vi "Enqueue.vi"(7 "Priority (F)":bool, 8 "错误输入（无错误）":errorcluster, 9 "Message Data":variant, 10 "Message":string, 11 "MessageQueue":refnum<queue>) -> (0 "error out":errorcluster, 3 "MessageQueue":refnum<queue>)   [LabVIEW 2019, in "module.lvlib"]
uses:
  module.lvlib
  Message.ctl
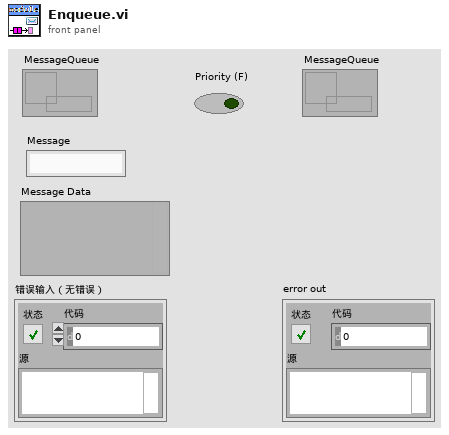
[diagram p1: front panel]
types:
  T1 = typedef "module.lvlib/Message.ctl" = cluster{"Message":string, "Message Data":variant}
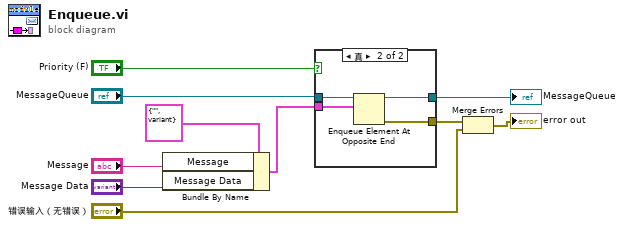
[diagram p0: block diagram]
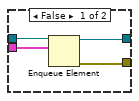
[diagram p2: hidden frame]
diagram:
  n1 = Bundle By Name(cluster=T1 {"Message"="", "Message Data"=variant} ("Message"), "Message"="Message", "Message Data"="Message Data") -> (w3:T1)
  n2 = case shown="真" "Priority (F)" {
    tunnel: "MessageQueue" -> [w14 w18]
    tunnel: [w12 w17] -> w7
    tunnel: [w13 w16] -> w9
    tunnel: w3 -> [w11 w15]
    frame False {
      n3 = Enqueue Element(queue=w14, element=w11) -> (queue out=w12:refnum<queue>, error out=w13:errorcluster)  [unwired: 2 in, 1 out]
    }
    frame True {
      n4 = Enqueue Element At Opposite End(queue=w18, element=w15) -> (queue out=w17:refnum<queue>, error out=w16:errorcluster)  [unwired: 2 in, 1 out]
    }
  }
  "MessageQueue" <- w7
  n5 = Merge Errors(w9, "错误输入（无错误）") -> (→"error out":errorcluster)
